vi "Stepper Read Position.vi"(2 "error in (no error)":errorcluster, 3 "Motor Number":u32=1 min=1 max=255 step=1, 4 "Instrument Address":refnum<visa-resource-name>) -> (0 "error out":errorcluster, 1 "Response":dbl format="%.2f")   [LabVIEW 2019]
uses:
  Parker Stepper Global.vi
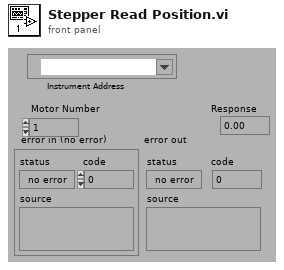
[diagram p1: front panel]
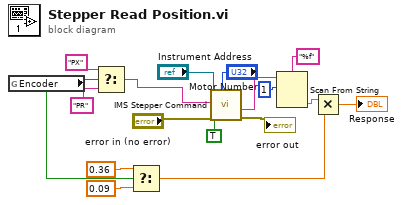
[diagram p0: block diagram]
diagram:
  n1 = global read "Parker Stepper Global.vi" "Encoder"() -> (w3:bool)
  n2 = Select(t="PX", s=w3, f="PR") -> (s? t:f=w6:string)
  n3 = Select(t=0.36 ("y"), s=w3, f=0.09 ("y")) -> (s? t:f=w1:dbl)
  n4 = call "IMS Stepper Command.vi"("Motor Number"="Motor Number", "error in (no error)"="error in (no error)", "Mode"=TRUE, "Command"=w6, "Instrument Address"="Instrument Address") -> ("error out"=→"error out":errorcluster, "Response"=w10:string)  [unwired: 1 in, 2 out]
  n5 = Scan From String(format string="%f", input string=w10, initial scan location=u32 1) -> (output 1=w12:dbl)  [unwired: 2 in, 3 out]
  n6 = Multiply(x=w12, y=w1) -> (x*y=→"Response":dbl)
